vi "I2C Write.vi"(5 "EOF":T1, 7 "I2C Channel (0)":u8, 8 "Error In":errorcluster, 9 "Data":u8[](array[numeric]), 10 "I2C Slave Address":u8, 11 "LINX Device Config":T2) -> (0 "Error Out":errorcluster, 3 "LINX Device Config":T2)   [LabVIEW 2014, in "LMH-LINX.lvlib" / "Device.lvlib"]
doc: "Write one or more bytes on the specified I2C channel."
uses:
  <vilib>/MakerHub/LINX/Private/Device/Device.lvlib
  <vilib>/MakerHub/LINX/Private/Device/Type Defs/LINX Device Config.ctl
  <vilib>/MakerHub/LINX/Private/Type Defs/Interface.ctl
  <vilib>/MakerHub/LINX/Private/Device/Type Defs/TCP Config.ctl
  <vilib>/MakerHub/LINX/Private/Device/Type Defs/Channels.ctl
  <vilib>/MakerHub/LINX/Private/Type Defs/Peripherals/I2C/EOF.ctl
  <vilib>/MakerHub/LINX/Private/Type Defs/Error Type.ctl
  <vilib>/MakerHub/LINX/LMH-LINX.lvlib
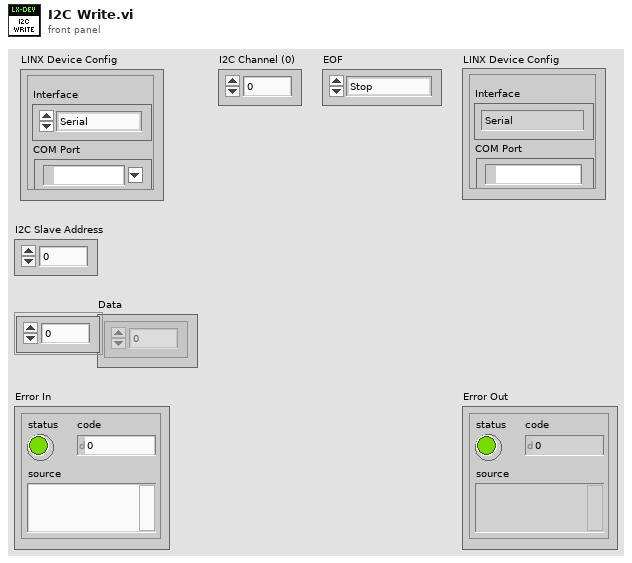
[diagram p1: front panel]
types:
  T1 = typedef "LMH-LINX.lvlib/EOF.ctl" = enum8{"Stop", "Restart", "Restart No Stop", "No Stop"}
  T2 = typedef "LMH-LINX.lvlib/Device.lvlib/LINX Device Config.ctl" = cluster{"Interface":T3, "COM Port":refnum<visa-resource-name>, "TCP Configuration":T4, "Device Family":u8, "Device ID":u8, "Device Name":string, "TCP Ref":refnum<k5>, "Channels":T5}
  T3 = typedef "LMH-LINX.lvlib/Interface.ctl" = enum16{"Serial", "TCP"}
  T4 = typedef "LMH-LINX.lvlib/Device.lvlib/TCP Config.ctl" = cluster{"IP Address":string, "Port":u16}
  T5 = typedef "LMH-LINX.lvlib/Channels.ctl" = cluster{"DI":u8[], "DO":u8[], "AI":u8[], "AO":u8[], "PWM":u8[], "QE":u8[], "UART":u8[], "I2C 2":u8[], "SPI":u8[], "CAN":u8[], "Servo":u8[], "AI Ref (V)":dbl, "AI Resolution (Bits)":u8, "AO Ref (V)":dbl, "AO Resolution (Bits)":u8}
  T6 = typedef "LMH-LINX.lvlib/Error Type.ctl" = enum16{"Unknown", "Timeout", "Corrupt Return Packet", "Unable To Connect", "Command Not Supported", "Channel DNE", "Invalid COM Config", "Firmware Version Mismatch", "myRIO Support", "CMD Specific Error", "Local IO Not Supported"}
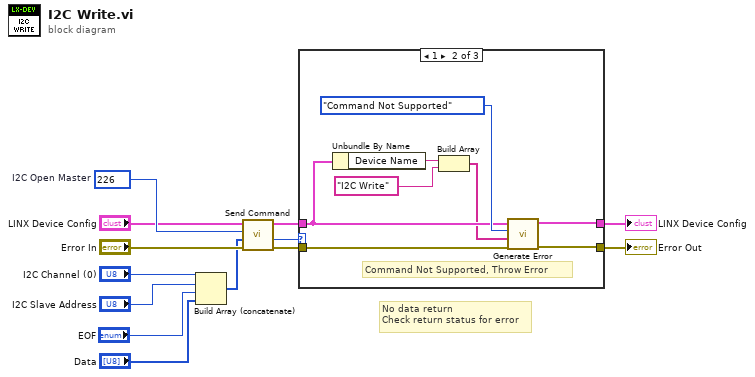
[diagram p0: block diagram]
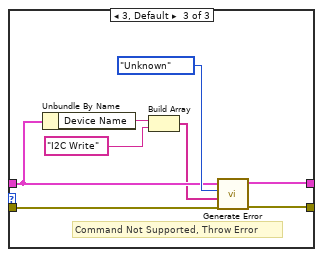
[diagram p3: hidden frame]
diagram:
  w12 = u16 226  # I2C Open Master
  # "No data return\nCheck return status for error"
  n1 = Build Array (concatenate)("I2C Channel (0)", "I2C Slave Address", "EOF", "Data") -> (w6:u8[])
  n2 = call <vilib>:"Send Command.vi"("Error In"="Error In", "ARGS"=w6, "CMD"=w12, "LINX Device Config"="LINX Device Config") -> ("Error Out"=w7:errorcluster, "Status"=w1:u8, "LINX Device Config"=w9:T2)  [unwired: 4 in, 1 out]
  n3 = case shown="1" w1 {
    tunnel: [w15 w21 w29] -> w10
    tunnel: w9 -> [w15 w19 w27]
    tunnel: [w14 w22 w30] -> w8
    tunnel: w7 -> [w14 w23 w31]
    frame 0 {
      # "Status OK, Process Data"
    }
    frame 1 {
      # "Command Not Supported, Throw Error"
      n4 = Unbundle By Name(w19) -> ("Device Name"=w18:string)
      n5 = Build Array(w18, "I2C Write") -> (w16:string[])
      n6 = call <vilib>:"Generate Error.vi"("Error In"=w23, "Arguments"=w16, "Error Type"=Error_Type."Command Not Supported", "LINX Device Config"=w19) -> ("Error Out"=w22:errorcluster, "Dup LINX Device Config"=w21:T2)  [unwired: 6 in]
    }
    frame 3, Default {
      # "Command Not Supported, Throw Error"
      n7 = Unbundle By Name(w27) -> ("Device Name"=w26:string)
      n8 = Build Array(w26, "I2C Write") -> (w24:string[])
      n9 = call <vilib>:"Generate Error.vi"("Error In"=w31, "Arguments"=w24, "Error Type"=Error_Type."Unknown", "LINX Device Config"=w27) -> ("Error Out"=w30:errorcluster, "Dup LINX Device Config"=w29:T2)  [unwired: 6 in]
    }
  }
  "Error Out" <- w8
  "LINX Device Config" <- w10
